vi "Read Sub Panel Msg.vi"(8 "error in (no error)":errorcluster, 11 "Msg in":refnum<class "Msg.lvclass">) -> (0 "error out":errorcluster, 2 "Sub Panel Msg":refnum<vi>, 3 "Msg out":refnum<class "Msg.lvclass">)   [LabVIEW 2020, in "Msg.lvlib" / "Msg.lvclass"]
uses:
  Msg.lvclass
  Msg.lvclass/Msg.ctl
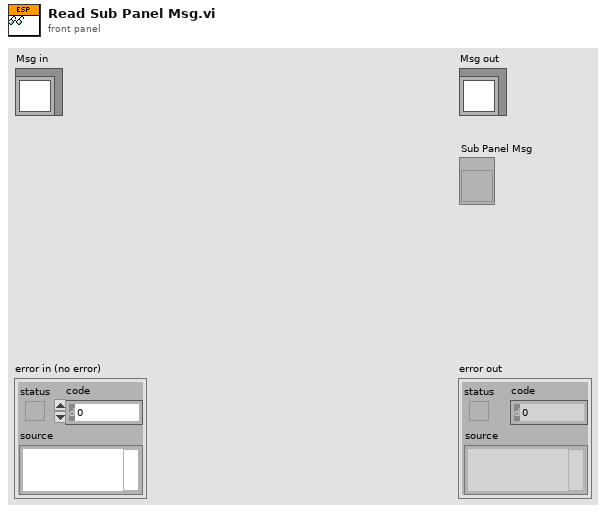
[diagram p1: front panel]
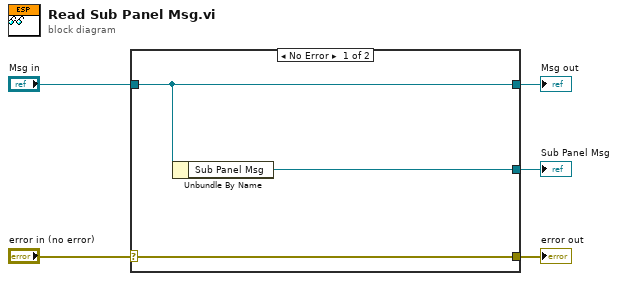
[diagram p0: block diagram]
diagram:
  n1 = case shown="No Error" "error in (no error)" {
    selector: "error in (no error)" -> [w8 w9]
    tunnel: [w8 w9] -> w4
    tunnel: [w7 w10] -> w2
    tunnel: "Msg in" -> [w7 w10]
    tunnel: [w6 _] -> w1
    frame No Error {
      n2 = Unbundle By Name(w7) -> ("Sub Panel Msg"=w6:refnum<vi>)
    }
    frame Error {
    }
  }
  "error out" <- w4
  "Msg out" <- w2
  "Sub Panel Msg" <- w1
